vi "Cosine Integral.vi"(3 "x":dbl format="%.2f") -> (1 "Ci(x)":dbl format="%.2f")   [LabVIEW 2010, in "NI_Gmath.lvlib"]
doc: "Evaluates the cosine integral for any real nonnegative number <B>x</B>."
uses:
  NI_Gmath.lvlib
  lvanlys.dll
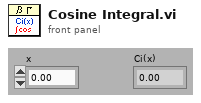
[diagram p1: front panel]
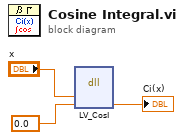
[diagram p0: block diagram]
diagram:
  n1 = dll-call lib="C:/Program Files/National Instruments/LabVIEW 2010/resource/lvanlys.*" fn="LV_CosI"("x"="x", "cosI(x)"=0.0 ("cosI")) -> ("cosI(x)"=→"Ci(x)":dbl)  [unwired: 5 in, 2 out]
